vi "MCCMSG Build Error Text.vi"(7 "uMaxLen":u32, 8 "error in (no error)":errorcluster, 9 "sTxtBuf":string, 10 "nErrorNum":i32, 11 "hMCCmsg":i32) -> (0 "error out":errorcluster, 1 "sTxtBuf out":string, 3 "function return":i32)   [LabVIEW 2012, in "MultiClamp 700B Controls.lvlib" / "AxMultiClampMsg.lvlib"]
doc: "AXMCCMSG BOOL WINAPI MCCMSG_BuildErrorText(HMCCMSG hMCCmsg, int nErrorNum, LPSTR sTxtBuf, UINT uMaxLen);"
uses:
  AxMultiClampMsg.lvlib
  AxMultiClampMsg.dll
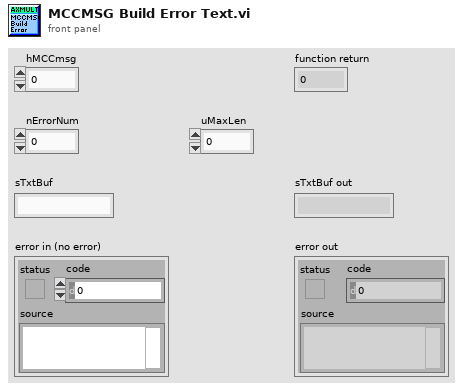
[diagram p1: front panel]
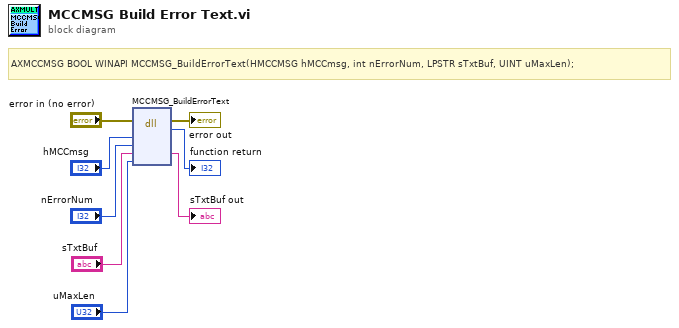
[diagram p0: block diagram]
diagram:
  # "AXMCCMSG BOOL WINAPI MCCMSG_BuildErrorText(HMCCMSG hMCCmsg, int nErrorNum, LPSTR sTxtBuf, UINT uMaxLen);"
  n1 = dll-call lib="C:/Users/Southampton/Desktop/Rita/Multiclamp 700B VIs/AxMultiClampMsg/AxMultiClampMsg.*" fn="MCCMSG_BuildErrorText"(error in="error in (no error)", "hMCCmsg"="hMCCmsg", "nErrorNum"="nErrorNum", "sTxtBuf"="sTxtBuf", "uMaxLen"="uMaxLen") -> (error out=→"error out":errorcluster, →"function return":i32, "sTxtBuf"=→"sTxtBuf out":string)  [unwired: 5 in, 1 out]
